vi "SMBus Write Word Protocol.vi"(4 "PEC":u8, 5 "Data":u16, 6 "CommandCode":u8, 7 "SlaveAddr":u8, 9 "SMBUSIndex":i32, 10 "DevIndex":i32, 11 "DevType":i32) -> (3 "function return":i32)   [LabVIEW 2010, in "ControlSMBus.lvlib"]
doc: "int WINAPI SMBus_WriteWordProtocol(int DevType,int DevIndex,int SMBUSIndex,unsigned char SlaveAddr,unsigned char CommandCode,unsigned short Data,unsigned char PEC);"
uses:
  ControlSMBus.lvlib
  ControlSMBus/Ginkgo_Driver.dll
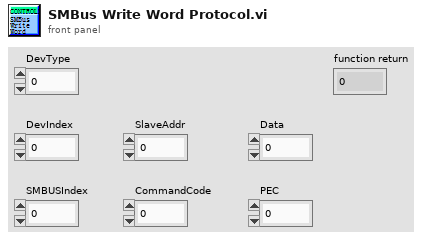
[diagram p1: front panel]
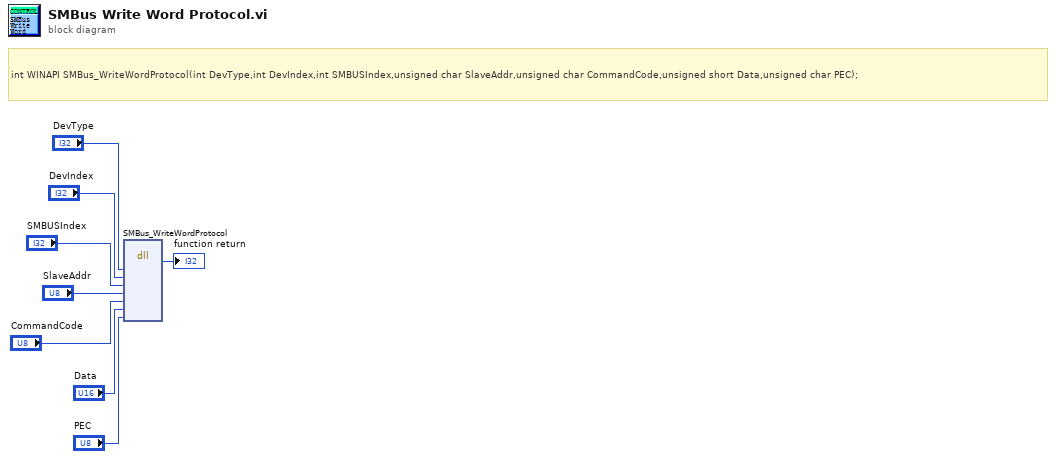
[diagram p0: block diagram]
diagram:
  # "int WINAPI SMBus_WriteWordProtocol(int DevType,int DevIndex,int SMBUSIndex,unsigned char SlaveAddr,unsigned char CommandCode,unsigned short Data,unsigned char PEC);"
  n1 = dll-call lib="E:/Project/vt_ginkgo/truck/Ginkgo Driver/vs2010/Ginkgo_USB-I2C&SPI&CAN_API_v2.0.3.3/lib/labview_32bit/ControlSMBus/Ginkgo_Driver.*" fn="SMBus_WriteWordProtocol"("DevType"="DevType", "DevIndex"="DevIndex", "SMBUSIndex"="SMBUSIndex", "SlaveAddr"="SlaveAddr", "CommandCode"="CommandCode", "Data"="Data", "PEC"="PEC") -> (→"function return":i32)  [unwired: 10 in, 2 out]
